vi "Slack-Get Bot.vi"(0 "config in":T1, 11 "error in (no error)":errorcluster) -> (4 "config out":T1, 15 "error out":errorcluster)   [LabVIEW 2020]
uses:
  Typedefs/Slack-Configuration.ctl
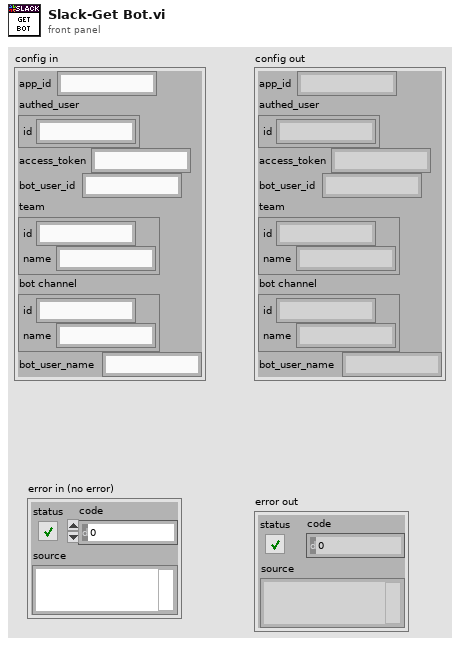
[diagram p1: front panel]
types:
  T1 = typedef "Slack-Configuration.ctl" = cluster{"app_id":string, "authed_user":cluster{"id":string}, "access_token":string, "bot_user_id":string, "team":cluster{"id":string, "name":string}, "bot channel":cluster{"id":string, "name":string}, "bot_user_name":string}
  T2 = typedef "Slack-User.ctl" = cluster{"id":string, "name":string}
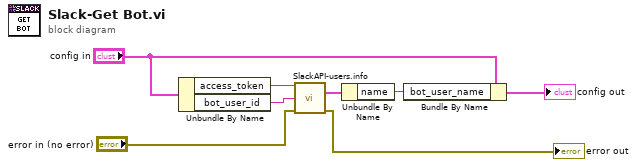
[diagram p0: block diagram]
diagram:
  n1 = Unbundle By Name("config in") -> ("access_token"=w7:string, "bot_user_id"=w8:string)
  n2 = call "SlackAPI-users.info.vi"("token"=w7, "user"=w8, "error in (no error)"="error in (no error)") -> ("user"=w5:T2, "error out"=→"error out":errorcluster)  [unwired: 10 in, 1 out]
  n3 = Unbundle By Name(w5) -> ("name"=w6:string)
  n4 = Bundle By Name(cluster="config in", "bot_user_name"=w6) -> (→"config out":T1)
